vi "1D_array_to_binary_data.vi"(7 "little-endian?":bool, 8 "error in (no error)":errorcluster, 11 "inputArray":variant) -> (0 "error out":errorcluster, 3 "BSONbytes":u8[](array[numeric]))   [LabVIEW 2015, in "BSON_convertors_Library.lvlib"]
doc: "Created by Artem Shevelev\nLabVIEW Portal profile: http://www.labviewportal.org/memberlist.php?mode=viewprofile&u=2340\ne-mail: artem.sh@gmail.com\nshevelev.pro"
uses:
  BSON_convertors_Library.lvlib
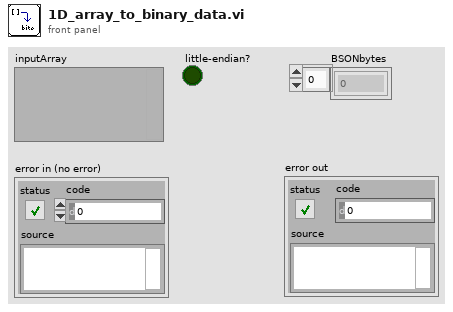
[diagram p1: front panel]
types:
  T1 = enum16{"big-endian, network order", "native, host order", "little-endian"}
  T2 = typedef "Type Descriptor Enumeration__ogtk.ctl" = enum8{"<Null>", "I8", "I16", "I32", "I64", "U8", "U16", "U32", "U64", "SGL", "DBL", "EXT", "CSG", "CDB", "CXT", "0x0F", "0x10", "0x11", "0x12", "0x13", "0x14", "Enum U8", "Enum U16", "Enum U32", "Enum U64", "SGL PQ", "DBL PQ", "EXT PQ", "CSG PQ", "CDB PQ", "CXT PQ", "0x1F", "0x20", "Boolean", "0x22", "0x23", "0x24", "0x25", "0x26", "0x27", "0x28", "0x29", "0x2A", "0x2B", "0x2C", "0x2D", "0x2E", "0x2F", "String", "0x31", "Path", "Pict", "0x34", "0x35", "0x36", "DAQ", "0x38", "0x39", "0x3A", "0x3B", "0x3C", "0x3D", "0x3E", "0x3F", "Array", "0x41", "0x42", "0x43", "0x44", "0x45", "0x46", "0x47", "0x48", "0x49", "0x4A", "0x4B", "0x4C", "0x4D", "0x4E", "0x4F", "Cluster", "0x51", "0x52", "Variant", "Waveform", "0x55", "0x56", "0x57", "0x58", "0x59", "0x5A", "0x5B", "0x5C", "0x5D", "0x5E", "0x5F", "0x60", "0x61", "0x62", "0x63", "0x64", "0x65", "0x66", "0x67", "0x68", "0x69", "0x6A", "0x6B", "0x6C", "0x6D", "0x6E", "0x6F", "Refnum"}
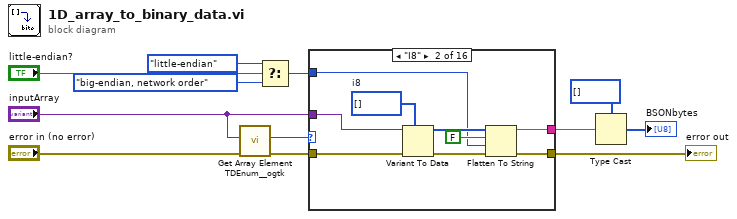
[diagram p0: block diagram]
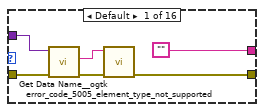
[diagram p2: hidden frame]
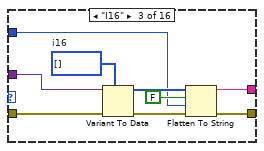
[diagram p3: hidden frame]
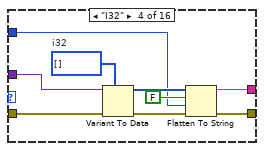
[diagram p4: hidden frame]
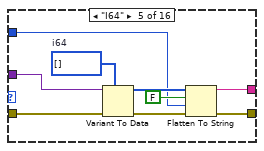
[diagram p5: hidden frame]
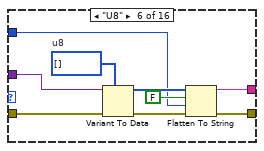
[diagram p6: hidden frame]
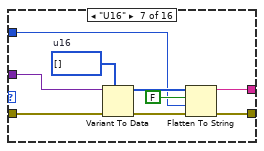
[diagram p7: hidden frame]
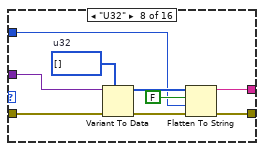
[diagram p8: hidden frame]
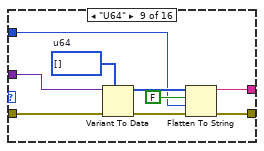
[diagram p9: hidden frame]
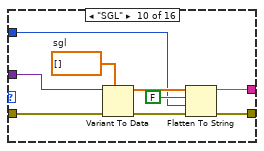
[diagram p10: hidden frame]
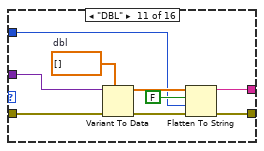
[diagram p11: hidden frame]
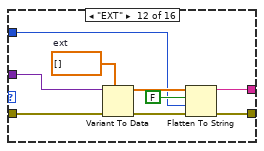
[diagram p12: hidden frame]
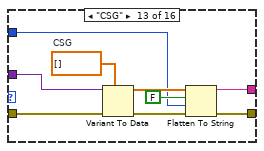
[diagram p13: hidden frame]
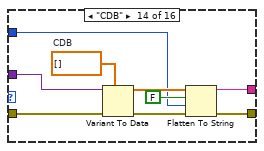
[diagram p14: hidden frame]
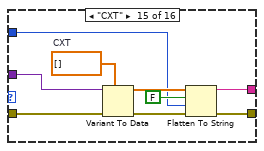
[diagram p15: hidden frame]
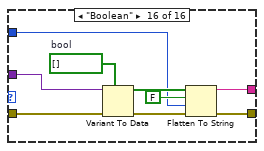
[diagram p16: hidden frame]
diagram:
  n1 = call <userlib>:"Get Array Element TDEnum__ogtk.vi"("error in (no error)"="error in (no error)", "Array"="inputArray") -> ("error out"=w3:errorcluster, "Element Type"=w2:T2)  [unwired: 8 in]
  n2 = Select(t=T1."little-endian" ("byte order (0:big-endian, network order)"), s="little-endian?", f=T1."big-endian, network order" ("byte order (0:big-endian, network order)")) -> (s? t:f=w9:T1)
  n3 = case shown="\"I8\"" w2 {
    tunnel: w3 -> [w16 w24 w33 w42 w51 w60 w69 w78 w87 w96 w105 w114 w123 w132 w141 w150]
    tunnel: "inputArray" -> [w18 w27 w36 w45 w54 w63 w72 w81 w90 w99 w108 w117 w126 w135 w144 w153]
    tunnel: [w14 w20 w29 w38 w47 w56 w65 w74 w83 w92 w101 w110 w119 w128 w137 w146] -> w5
    tunnel: w9 -> [_ w21 w30 w39 w48 w57 w66 w75 w84 w93 w102 w111 w120 w129 w138 w147]
    tunnel: ["" w19 w28 w37 w46 w55 w64 w73 w82 w91 w100 w109 w118 w127 w136 w145] -> w11
    frame Default {
      n4 = call <userlib>:"Get Data Name__ogtk.vi"("error in (no error)"=w16, "Data"=w18) -> ("error out"=w15:errorcluster, "Data Name"=w17:string)  [unwired: 7 in, 1 out]
      n5 = call "error_code_5005_element_type_not_supported.vi"("error in (no error)"=w15, "name"=w17) -> ("error out"=w14:errorcluster)  [unwired: 9 in]
    }
    frame "I8" {
      w26 = i8[] []  # i8
      n6 = Variant To Data(error in=w24, type=w26, Variant=w27) -> (data=w25:i8[], error out=w23:errorcluster)
      n7 = Flatten To String(anything=w25, prepend array or string size? (T)=FALSE, byte order (0:big-endian, network order)=w21, error in (no error)=w23) -> (data string=w19:string, error out=w20:errorcluster)  [unwired: 1 out]
    }
    frame "I16" {
      w35 = i16[] []  # i16
      n8 = Variant To Data(error in=w33, type=w35, Variant=w36) -> (data=w34:i16[], error out=w32:errorcluster)
      n9 = Flatten To String(anything=w34, prepend array or string size? (T)=FALSE, byte order (0:big-endian, network order)=w30, error in (no error)=w32) -> (data string=w28:string, error out=w29:errorcluster)  [unwired: 1 out]
    }
    frame "I32" {
      w44 = i32[] []  # i32
      n10 = Variant To Data(error in=w42, type=w44, Variant=w45) -> (data=w43:i32[], error out=w41:errorcluster)
      n11 = Flatten To String(anything=w43, prepend array or string size? (T)=FALSE, byte order (0:big-endian, network order)=w39, error in (no error)=w41) -> (data string=w37:string, error out=w38:errorcluster)  [unwired: 1 out]
    }
    frame "I64" {
      w53 = i64[] []  # i64
      n12 = Variant To Data(error in=w51, type=w53, Variant=w54) -> (data=w52:i64[], error out=w50:errorcluster)
      n13 = Flatten To String(anything=w52, prepend array or string size? (T)=FALSE, byte order (0:big-endian, network order)=w48, error in (no error)=w50) -> (data string=w46:string, error out=w47:errorcluster)  [unwired: 1 out]
    }
    frame "U8" {
      w62 = u8[] []  # u8
      n14 = Variant To Data(error in=w60, type=w62, Variant=w63) -> (data=w61:u8[], error out=w59:errorcluster)
      n15 = Flatten To String(anything=w61, prepend array or string size? (T)=FALSE, byte order (0:big-endian, network order)=w57, error in (no error)=w59) -> (data string=w55:string, error out=w56:errorcluster)  [unwired: 1 out]
    }
    frame "U16" {
      w71 = u16[] []  # u16
      n16 = Variant To Data(error in=w69, type=w71, Variant=w72) -> (data=w70:u16[], error out=w68:errorcluster)
      n17 = Flatten To String(anything=w70, prepend array or string size? (T)=FALSE, byte order (0:big-endian, network order)=w66, error in (no error)=w68) -> (data string=w64:string, error out=w65:errorcluster)  [unwired: 1 out]
    }
    frame "U32" {
      w80 = u32[] []  # u32
      n18 = Variant To Data(error in=w78, type=w80, Variant=w81) -> (data=w79:u32[], error out=w77:errorcluster)
      n19 = Flatten To String(anything=w79, prepend array or string size? (T)=FALSE, byte order (0:big-endian, network order)=w75, error in (no error)=w77) -> (data string=w73:string, error out=w74:errorcluster)  [unwired: 1 out]
    }
    frame "U64" {
      w89 = u64[] []  # u64
      n20 = Variant To Data(error in=w87, type=w89, Variant=w90) -> (data=w88:u64[], error out=w86:errorcluster)
      n21 = Flatten To String(anything=w88, prepend array or string size? (T)=FALSE, byte order (0:big-endian, network order)=w84, error in (no error)=w86) -> (data string=w82:string, error out=w83:errorcluster)  [unwired: 1 out]
    }
    frame "SGL" {
      w98 = sgl[] []  # sgl
      n22 = Variant To Data(error in=w96, type=w98, Variant=w99) -> (data=w97:sgl[], error out=w95:errorcluster)
      n23 = Flatten To String(anything=w97, prepend array or string size? (T)=FALSE, byte order (0:big-endian, network order)=w93, error in (no error)=w95) -> (data string=w91:string, error out=w92:errorcluster)  [unwired: 1 out]
    }
    frame "DBL" {
      w107 = dbl[] []  # dbl
      n24 = Variant To Data(error in=w105, type=w107, Variant=w108) -> (data=w106:dbl[], error out=w104:errorcluster)
      n25 = Flatten To String(anything=w106, prepend array or string size? (T)=FALSE, byte order (0:big-endian, network order)=w102, error in (no error)=w104) -> (data string=w100:string, error out=w101:errorcluster)  [unwired: 1 out]
    }
    frame "EXT" {
      w116 = ext[] []  # ext
      n26 = Variant To Data(error in=w114, type=w116, Variant=w117) -> (data=w115:ext[], error out=w113:errorcluster)
      n27 = Flatten To String(anything=w115, prepend array or string size? (T)=FALSE, byte order (0:big-endian, network order)=w111, error in (no error)=w113) -> (data string=w109:string, error out=w110:errorcluster)  [unwired: 1 out]
    }
    frame "CSG" {
      w125 = csg[] []  # CSG
      n28 = Variant To Data(error in=w123, type=w125, Variant=w126) -> (data=w124:csg[], error out=w122:errorcluster)
      n29 = Flatten To String(anything=w124, prepend array or string size? (T)=FALSE, byte order (0:big-endian, network order)=w120, error in (no error)=w122) -> (data string=w118:string, error out=w119:errorcluster)  [unwired: 1 out]
    }
    frame "CDB" {
      w134 = cdb[] []  # CDB
      n30 = Variant To Data(error in=w132, type=w134, Variant=w135) -> (data=w133:cdb[], error out=w131:errorcluster)
      n31 = Flatten To String(anything=w133, prepend array or string size? (T)=FALSE, byte order (0:big-endian, network order)=w129, error in (no error)=w131) -> (data string=w127:string, error out=w128:errorcluster)  [unwired: 1 out]
    }
    frame "CXT" {
      w143 = cxt[] []  # CXT
      n32 = Variant To Data(error in=w141, type=w143, Variant=w144) -> (data=w142:cxt[], error out=w140:errorcluster)
      n33 = Flatten To String(anything=w142, prepend array or string size? (T)=FALSE, byte order (0:big-endian, network order)=w138, error in (no error)=w140) -> (data string=w136:string, error out=w137:errorcluster)  [unwired: 1 out]
    }
    frame "Boolean" {
      w152 = bool[] []  # bool
      n34 = Variant To Data(error in=w150, type=w152, Variant=w153) -> (data=w151:bool[], error out=w149:errorcluster)
      n35 = Flatten To String(anything=w151, prepend array or string size? (T)=FALSE, byte order (0:big-endian, network order)=w147, error in (no error)=w149) -> (data string=w145:string, error out=w146:errorcluster)  [unwired: 1 out]
    }
  }
  "error out" <- w5
  n36 = Type Cast(type=u8[] [] ("BSONbytes"), x=w11) -> (*(type *) &x=→"BSONbytes":u8[])
